vi "FeedbackDecode_MSMS2DEKA.vi"(7 "CtrlMode":T1(array[ring])=[enum."Position", enum."Position", enum."Position", enum."Position", enum."Position", enum."Position", enum."Position", enum."Position", enum."Position", enum."Position", enum."Position", enum."Position"], 8 "Sensors":T3={"Position"={"WriRot"=-84.0, "WriPitch"=-163.0, "IndFlex"=3175.0, "MRPFlex"=2598.0, "ThuRawPitch"=2802.0, "ThuRawYaw"=4899.0, "ThuYaw"=1941.0, "ThuPitch"=4899.0}, "Force"={"IndLat"=20.0, "IndTip"=36.0, "MidTip"=27.0, "RinTip"=34.0, "PinkyTip"=24.0, "PalmDist"=57.0, "PalmProx"=68.0, "HandEdge"=25.0, "HandDorsal"=105.0, "ThuUlnar"=15.0, "ThuRadial"=15.0, "ThuTip"=14.0, "ThuDorsal"=21.0}}, 9 "ConnDEKA":bool, 10 "ResetPID":bool, 11 "MSMSMvnt":dbl[](array[numeric])=[0.0, 0.0, 0.0, 0.0, 0.0, 0.0, 0.0, 0.0, 0.0, 0.0, 0.0, 0.0] min=-1.0 max=1.0) -> (0 "ACIOut":T4[](array[typedef])=[{"Timestamp"=0.0, "ArbitrationId"=528, "IsRemote"=0, "DataLength"=8, "Data"=[0, 0, 0, 0, 0, 38, 0, 0]}, {"Timestamp"=0.0, "ArbitrationId"=529, "IsRemote"=0, "DataLength"=8, "Data"=[0, 0, 0, 52, 0, 50, 0, 0]}, {"Timestamp"=0.0, "ArbitrationId"=530, "IsRemote"=0, "DataLength"=8, "Data"=[0, 26, 0, 0, 0, 0, 0, 47]}, {"Timestamp"=0.0, "ArbitrationId"=531, "IsRemote"=0, "DataLength"=8, "Data"=[0, 0, 0, 0, 0, 0, 0, 0]}] {"Data" format="%.0x"; "ArbitrationId" format="%.0x"; "Timestamp" format="%<%I:%M:%S%3u %p\n%m/%d/%Y>T"})   [LabVIEW 2020]
uses:
  <vilib>/nican/nican.llb/CanFrameTimed.ctl
  <vilib>/addons/control/pid/pid.llb/PID Advanced (DBL Array).vi
  <vilib>/addons/control/pid/pid.llb/PID Parameter Manager (DBL Array).vi
  <vilib>/addons/control/pid/pid.llb/PID Derivative Action Buffered (DBL Array).vi
  <vilib>/addons/control/pid/pid.llb/PID Get Advanced Error (DBL Array).vi
  <vilib>/addons/control/pid/pid.llb/PID Integral Action Buffered (DBL Array).vi
  <vilib>/addons/control/pid/pid.llb/PID Resize 1D Array.vi
  <vilib>/addons/control/pid/pid.llb/PID Get Advanced Error (DBL).vi
  FeedbackDecode_Globals.vi
  <vilib>/addons/control/pid/pid.llb/PID Output Rate Limiter (DBL Array).vi
  <vilib>/addons/control/pid/NI_PID_pid.lvlib
panel:
  in  "HandType":enum16{"Left", "Right"}(ring)=enum."Right"
  in  "SetPoint":dbl[](array[numeric])=[0.85, 0.35, 0.35, 0.35, 0.0, 0.0]
  in  "RmThresh":dbl
  in  "ThuMin":dbl=4000.0
  in  "ThuMax":dbl=5800.0
  in  "linearity":dbl=1.0 format="%.2f"
  in  "outputrate":dbl=3000.0 format="%.2f"
  in  "PIDGains":T2(array[cluster])=[{"proportional gain (Kc)"=0.5, "integral time (Ti, min)"=0.0, "derivative time (Td, min)"=0.0}, {"proportional gain (Kc)"=1.0, "integral time (Ti, min)"=0.0, "derivative time (Td, min)"=0.0}, {"proportional gain (Kc)"=1.0, "integral time (Ti, min)"=0.0, "derivative time (Td, min)"=0.0}, {"proportional gain (Kc)"=1.0, "integral time (Ti, min)"=0.0, "derivative time (Td, min)"=0.0}, {"proportional gain (Kc)"=3.0, "integral time (Ti, min)"=0.0, "derivative time (Td, min)"=0.0}, {"proportional gain (Kc)"=3.0, "integral time (Ti, min)"=0.0, "derivative time (Td, min)"=0.0}] {"derivative time (Td, min)" format="%.5f"; "integral time (Ti, min)" format="%.5f"; "proportional gain (Kc)" format="%.5f"}
  in  "ACIInit":T4[](array[typedef])=[{"Timestamp"=0.0, "ArbitrationId"=528, "IsRemote"=0, "DataLength"=8, "Data"=[0, 0, 0, 0, 0, 0, 0, 0]}, {"Timestamp"=0.0, "ArbitrationId"=529, "IsRemote"=0, "DataLength"=8, "Data"=[0, 0, 0, 0, 0, 0, 0, 0]}, {"Timestamp"=0.0, "ArbitrationId"=530, "IsRemote"=0, "DataLength"=8, "Data"=[0, 0, 0, 0, 0, 0, 0, 0]}, {"Timestamp"=0.0, "ArbitrationId"=531, "IsRemote"=0, "DataLength"=8, "Data"=[0, 0, 0, 0, 0, 0, 0, 0]}] {"Data" format="%.0x"; "ArbitrationId" format="%.0x"; "Timestamp" format="%<%I:%M:%S%3u %p\n%m/%d/%Y>T"}
  # "ThuLimit of 5800 aligns with index,\n~6000 for tripod."
  # "ThuPitch"
  # "Thumb"
  # "Index"
  # "Middle"
  # "ThuYaw"
  # "Ring"
  # "Little"
  # "ThumbInt"
  # "ThuPitchUp"
  # "IndFlex"
  # "IndexInt"
  # "ThuPitchDown"
  # "Ring Int"
  # "ThuYawRight"
  # "Little Int"
  # "ThuYawLeft"
  # "WristPitch"
  # "MRPFlex"
  # "WristYaw"
  # "IndFlex"
  # "WristRoll"
  # "IndExt"
  # "WriRot"
  # "MRPFlex"
  # "MRPExt"
  # "WriPitch"
  # "WriPronate"
  # "WriSupinate"
  # "WriExt"
  # "WriFlex"
  # "ModeSelect"
  # "N/A"
  # "N/A"
  # "N/A"
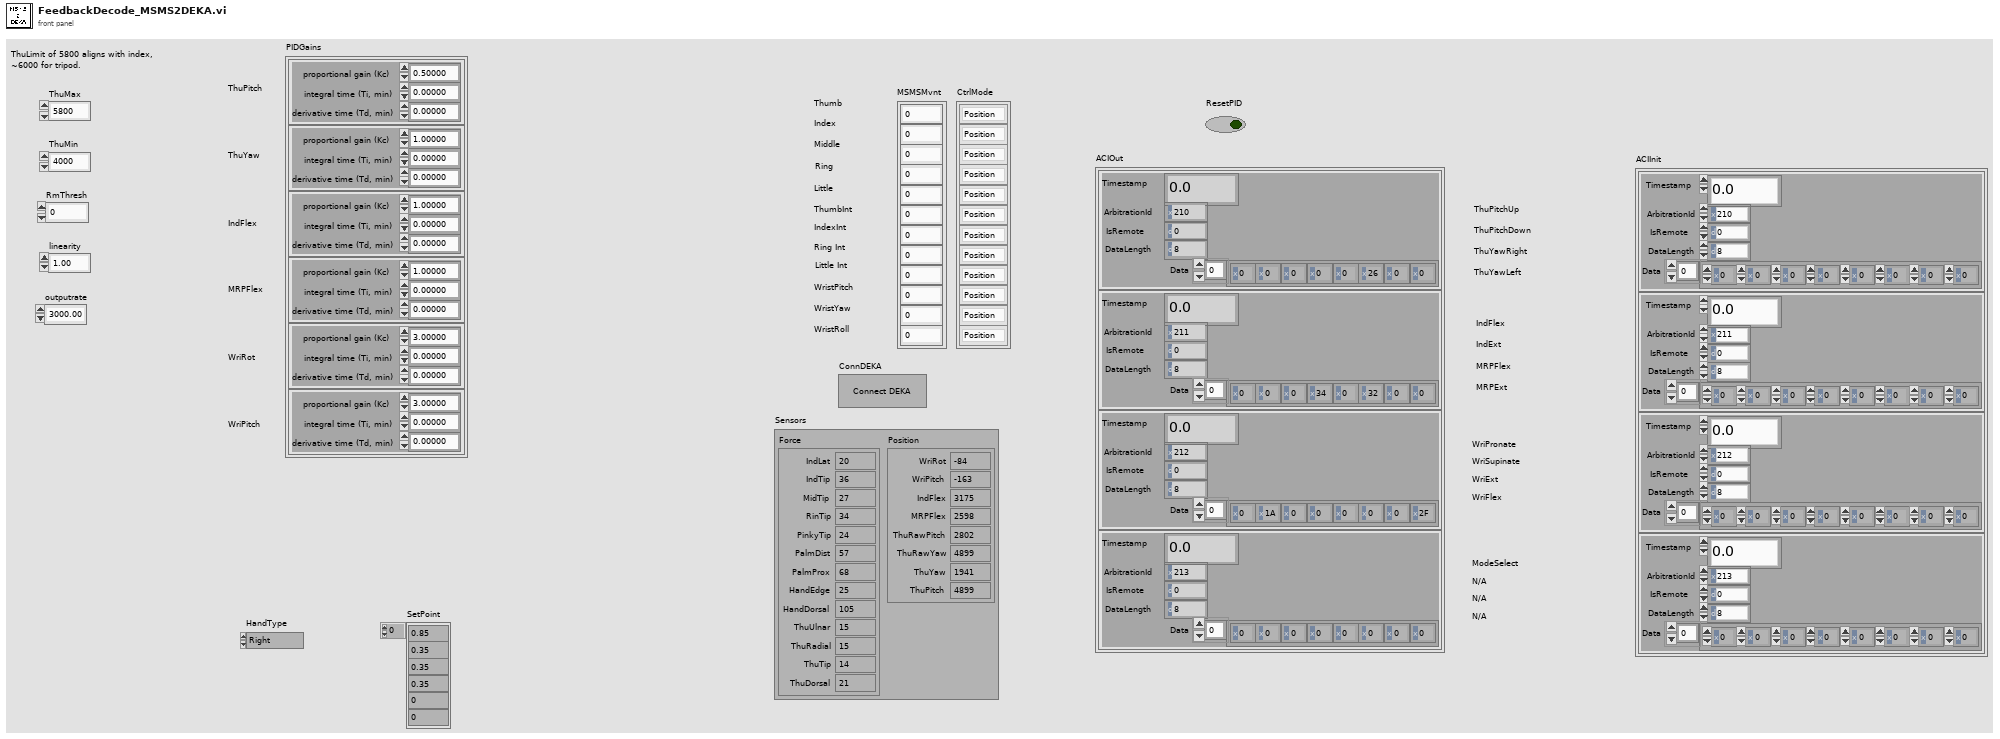
[diagram p1: front panel]
types:
  T1 = enum16{"Position", "Latching", "Leaky", "Velocity"}[]
  T2 = cluster{"proportional gain (Kc)":dbl, "integral time (Ti, min)":dbl, "derivative time (Td, min)":dbl}[]
  T3 = cluster{"Position":cluster{"WriRot":dbl, "WriPitch":dbl, "IndFlex":dbl, "MRPFlex":dbl, "ThuRawPitch":dbl, "ThuRawYaw":dbl, "ThuYaw":dbl, "ThuPitch":dbl}, "Force":cluster{"IndLat":dbl, "IndTip":dbl, "MidTip":dbl, "RinTip":dbl, "PinkyTip":dbl, "PalmDist":dbl, "PalmProx":dbl, "HandEdge":dbl, "HandDorsal":dbl, "ThuUlnar":dbl, "ThuRadial":dbl, "ThuTip":dbl, "ThuDorsal":dbl}}
  T4 = typedef "CanFrameTimed.ctl" = cluster{"Timestamp":dbl, "ArbitrationId":u32, "IsRemote":u8, "DataLength":u8, "Data":u8[]}
  T5 = cluster{"setpoint high":dbl, "setpoint low":dbl}[]
  T6 = enum16{"Position", "Latching", "Leaky", "Velocity"}
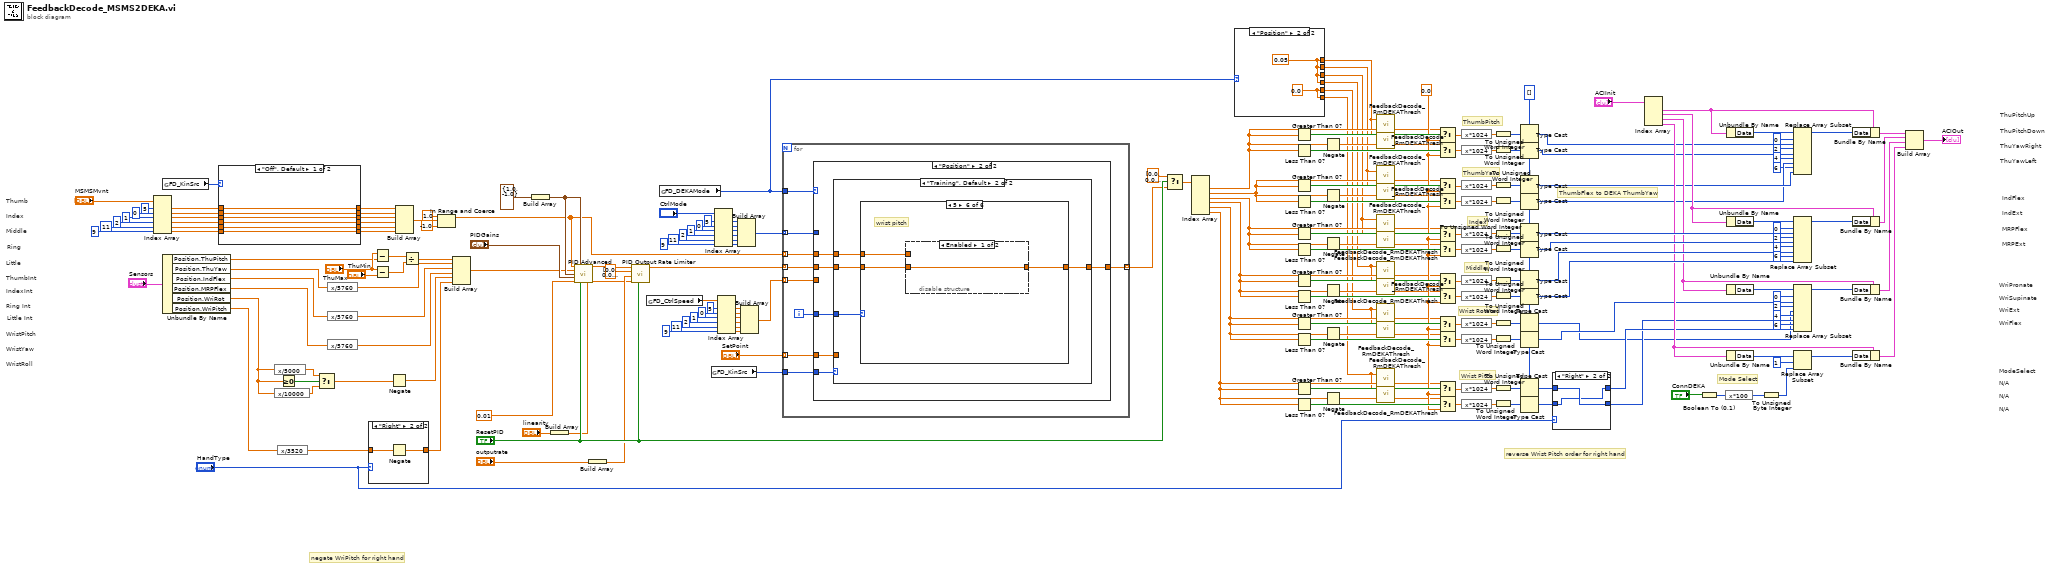
[diagram p0: block diagram]
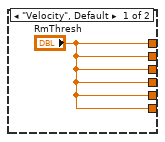
[diagram p4: hidden frame]
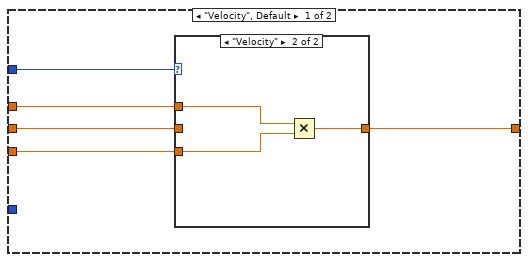
[diagram p5: hidden frame]
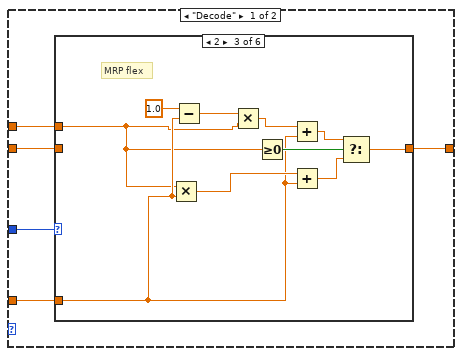
[diagram p7: hidden frame]
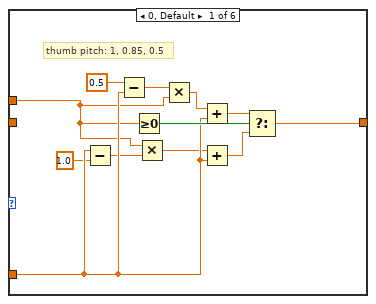
[diagram p8: hidden frame]
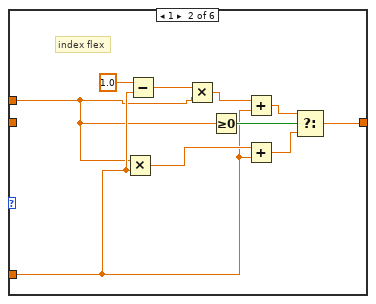
[diagram p9: hidden frame]
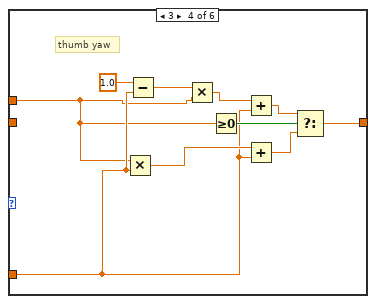
[diagram p10: hidden frame]
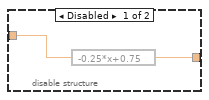
[diagram p14: hidden frame]
diagram:
  w144 = u8[] []
  w86 = 0.0
  # "reverse Wrist Pitch order for right hand"
  # "negate WriPitch for right hand"
  # "ThumbPitch"
  # "N/A"
  # "N/A"
  # "N/A"
  # "ModeSelect"
  # "WriFlex"
  # "WriExt"
  # "WriSupinate"
  # "WriPronate"
  # "MRPExt"
  # "MRPFlex"
  # "IndExt"
  # "IndFlex"
  # "ThuYawLeft"
  # "ThuYawRight"
  # "ThuPitchDown"
  # "ThuPitchUp"
  # "ThumbFlex to DEKA ThumbYaw"
  # "Mode Select"
  # "Wrist Pitch"
  # "Wrist Rotate"
  # "Middle"
  # "Index"
  # "ThumbYaw"
  # "Little Int"
  # "WristRoll"
  # "WristYaw"
  # "WristPitch"
  # "Ring Int"
  # "IndexInt"
  # "ThumbInt"
  # "Little"
  # "Ring"
  # "Middle"
  # "Index"
  # "Thumb"
  n1 = Index Array(array="MSMSMvnt", index #1=5 ("index"), index #2=0 ("index"), index #3=1 ("index"), index #4=2 ("index"), index #5=11 ("index"), index #6=9 ("index")) -> (element #1=w60:dbl, element #2=w59:dbl, element #3=w58:dbl, element #4=w57:dbl, element #5=w56:dbl, element #6=w55:dbl)
  n2 = global read "FeedbackDecode_Globals.vi" "FD_KinSrc"() -> (w61:enum16{"Off", "Training", "Decode", "COB"})
  n3 = Unbundle By Name("Sensors") -> ("Position.ThuPitch"=w95:dbl, "Position.ThuYaw"=w133:dbl, "Position.IndFlex"=w132:dbl, "Position.MRPFlex"=w131:dbl, "Position.WriRot"=w106:dbl, "Position.WriPitch"=w5:dbl)
  n4 = case shown="\"Off\", Default" w61 {
    tunnel: w60 -> [w230 w238]
    tunnel: w59 -> [w229 w236]
    tunnel: w58 -> [w228 w234]
    tunnel: w57 -> [w227 w232]
    tunnel: w56 -> [w226 w240]
    tunnel: w55 -> [w225 w239]
    tunnel: [w230 w237] -> w54
    tunnel: [w229 w235] -> w53
    tunnel: [w228 w233] -> w52
    tunnel: [w227 w231] -> w51
    tunnel: [w226 w240] -> w50
    tunnel: [w225 w239] -> w49
    frame "Off", Default {
    }
    frame "Training" {
      n5 = expression code="x*0.5+0.5"(w238) -> (w237:dbl)
      n6 = expression code="x*0.5+0.3"(w236) -> (w235:dbl)
      n7 = expression code="x*0.5+0.5"(w234) -> (w233:dbl)
      n8 = expression code="x*0.5+0.5"(w232) -> (w231:dbl)
    }
  }
  n9 = expression code="x/5000"(w106) -> (w108:dbl)
  n10 = expression code="x/10000"(w106) -> (w107:dbl)
  n11 = expression code="x/3520"(w5) -> (w4:dbl)
  n12 = Greater Or Equal To 0?(x=w106) -> (x >= 0?=w109:bool)
  n13 = Select(t=w108, s=w109, f=w107) -> (s? t:f=w3:dbl)
  n14 = expression code="x/5760"(w133) -> (w103:dbl)
  n15 = expression code="x/5760"(w132) -> (w102:dbl)
  n16 = expression code="x/5760"(w131) -> (w101:dbl)
  n17 = case shown="\"Right\"" "HandType" {
    tunnel: w4 -> [w241 w242]
    tunnel: [w241 w243] -> w100
    frame "Left", Default {
    }
    frame "Right" {
      n18 = Negate(x=w242) -> (-x=w243:dbl)
    }
  }
  n19 = Subtract(x="ThuMax", y=w95) -> (x-y=w97:dbl)
  n20 = Subtract(x="ThuMax", y="ThuMin") -> (x-y=w96:dbl)
  n21 = Negate(x=w3) -> (-x=w2:dbl)
  n22 = Build Array(w54, w53, w52, w51, w50, w49) -> (w123:dbl[])
  n23 = Divide(x=w97, y=w96) -> (x/y=w94:dbl)
  n24 = In Range and Coerce(upper limit=1.0, x=w123, lower limit=-1.0) -> (coerced(x)=w110:dbl[])  [unwired: 1 out]
  n25 = Build Array(w94, w103, w102, w101, w2, w100) -> (w99:dbl[])
  n26 = Build Array(cluster{"setpoint high":dbl, "setpoint low":dbl} {"setpoint high"=1.0, "setpoint low"=-1.0} ("setpoint range")) -> (w113:T5)
  n27 = Build Array("linearity") -> (w114:dbl[])
  n28 = call-poly <vilib>:"PID Advanced.vi"("setpoint"=w110, "output range"=w113, "process variable"=w99, "setpoint range"=w113, "PID gains"="PIDGains", "dt (s)"=0.01, "reinitialize? (F)"="ResetPID", "linearity"=w114) -> ("output"=w119:dbl[], "dt out (s)"=w116:dbl)  [unwired: 6 in]
  n29 = Build Array("outputrate") -> (w117:dbl[])
  n30 = call-poly <vilib>:"PID Output Rate Limiter.vi"("reinitialize? (F)"="ResetPID", "dt (s)"=w116, "output rate (EGU/min)"=w117, "initial output"=dbl[] [0.0, 0.0, 0.0, 0.0, 0.0, 0.0], "input (controller output)"=w119) -> ("output"=w112:dbl[])  [unwired: 3 in, 1 out]
  n31 = global read "FeedbackDecode_Globals.vi" "FD_CtrlSpeed"() -> (w22:sgl[])
  n32 = global read "FeedbackDecode_Globals.vi" "FD_DEKAMode"() -> (w20:enum16{"Velocity", "Position"})
  n33 = global read "FeedbackDecode_Globals.vi" "FD_KinSrc"() -> (w13:enum16{"Off", "Training", "Decode", "COB"})
  n34 = Index Array(array="CtrlMode", index #1=5 ("index"), index #2=0 ("index"), index #3=1 ("index"), index #4=2 ("index"), index #5=11 ("index"), index #6=9 ("index")) -> (element #1=w41:T6, element #2=w40:T6, element #3=w39:T6, element #4=w38:T6, element #5=w37:T6, element #6=w36:T6)
  n35 = Index Array(array=w22, index #1=5 ("index"), index #2=0 ("index"), index #3=1 ("index"), index #4=2 ("index"), index #5=11 ("index"), index #6=9 ("index")) -> (element #1=w29:sgl, element #2=w30:sgl, element #3=w31:sgl, element #4=w32:sgl, element #5=w33:sgl, element #6=w34:sgl)
  n36 = Build Array(w41, w40, w39, w38, w37, w36) -> (w35:T1)
  n37 = Build Array(w29, w30, w31, w32, w33, w34) -> (w21:sgl[])
  n38 = for {
    tunnel: w112 -> [w252] mode=indexing
    tunnel: [w251] -> w111 mode=indexing
    tunnel: w110 -> [w250] mode=indexing
    tunnel: w35 -> [w249] mode=indexing
    tunnel: w21 -> [w248] mode=indexing
    tunnel: w20 -> [w247]
    tunnel: w13 -> [w245]
    tunnel: "SetPoint" -> [w244] mode=indexing
    i -> [w246]
    n39 = case shown="\"Position\"" w247 {
      tunnel: w252 -> [w257 w264]
      tunnel: [w256 w265] -> w251
      tunnel: w250 -> [w255 w266]
      tunnel: w249 -> [w254 _]
      tunnel: w248 -> [w253 _]
      tunnel: w246 -> [_ w267]
      tunnel: w245 -> [_ w263]
      tunnel: w244 -> [_ w262]
      frame "Velocity", Default {
        n40 = case shown="\"Velocity\"" w254 {
          tunnel: w257 -> [w258 _]
          tunnel: [w258 w260] -> w256
          tunnel: w255 -> [_ w261]
          tunnel: w253 -> [_ w259]
          frame "Position", Default {
          }
          frame "Velocity" {
            n41 = Multiply(x=w261, y=w259) -> (x*y=w260:dbl)
          }
        }
      }
      frame "Position" {
        n42 = case shown="\"Training\", Default" w263 {
          tunnel: w267 -> [w272 w317]
          tunnel: w266 -> [w271 w320]
          tunnel: [w270 w319] -> w265
          tunnel: w264 -> [w269 w318]
          tunnel: w262 -> [w268 _]
          frame "Decode" {
            n43 = case shown="2" w272 {
              tunnel: w271 -> [w274 w286 w296 w306 _ _]
              tunnel: [w283 w293 w303 w313 w315 w316] -> w270
              tunnel: w269 -> [_ _ _ _ w315 w316]
              tunnel: w268 -> [w277 w288 w298 w308 _ _]
              frame 0, Default {
                # "thumb pitch: 1, 0.85, 0.5"
                n44 = Subtract(x=w277, y=1.0) -> (x-y=w275:dbl)
                n45 = Subtract(x=0.5, y=w277) -> (x-y=w279:dbl)
                n46 = Greater Or Equal To 0?(x=w274) -> (x >= 0?=w284:bool)
                n47 = Multiply(x=w274, y=w275) -> (x*y=w273:dbl)
                n48 = Multiply(x=w279, y=w274) -> (x*y=w278:dbl)
                n49 = Add(x=w278, y=w277) -> (x+y=w281:dbl)
                n50 = Add(x=w273, y=w277) -> (x+y=w282:dbl)
                n51 = Select(t=w281, s=w284, f=w282) -> (s? t:f=w283:dbl)
              }
              frame 1 {
                # "index flex"
                n52 = Multiply(x=w286, y=w288) -> (x*y=w290:dbl)
                n53 = Subtract(x=1.0, y=w288) -> (x-y=w287:dbl)
                n54 = Multiply(x=w287, y=w286) -> (x*y=w285:dbl)
                n55 = Greater Or Equal To 0?(x=w286) -> (x >= 0?=w294:bool)
                n56 = Add(x=w285, y=w288) -> (x+y=w292:dbl)
                n57 = Add(x=w290, y=w288) -> (x+y=w291:dbl)
                n58 = Select(t=w292, s=w294, f=w291) -> (s? t:f=w293:dbl)
              }
              frame 2 {
                # "MRP flex"
                n59 = Multiply(x=w296, y=w298) -> (x*y=w300:dbl)
                n60 = Subtract(x=1.0, y=w298) -> (x-y=w297:dbl)
                n61 = Multiply(x=w297, y=w296) -> (x*y=w295:dbl)
                n62 = Greater Or Equal To 0?(x=w296) -> (x >= 0?=w304:bool)
                n63 = Add(x=w295, y=w298) -> (x+y=w302:dbl)
                n64 = Add(x=w300, y=w298) -> (x+y=w301:dbl)
                n65 = Select(t=w302, s=w304, f=w301) -> (s? t:f=w303:dbl)
              }
              frame 3 {
                # "thumb yaw"
                n66 = Multiply(x=w306, y=w308) -> (x*y=w310:dbl)
                n67 = Subtract(x=1.0, y=w308) -> (x-y=w307:dbl)
                n68 = Multiply(x=w307, y=w306) -> (x*y=w305:dbl)
                n69 = Greater Or Equal To 0?(x=w306) -> (x >= 0?=w314:bool)
                n70 = Add(x=w305, y=w308) -> (x+y=w312:dbl)
                n71 = Add(x=w310, y=w308) -> (x+y=w311:dbl)
                n72 = Select(t=w312, s=w314, f=w311) -> (s? t:f=w313:dbl)
              }
              frame 4 {
                # "wrist rotation"
              }
              frame 5 {
                # "wrist pitch"
              }
            }
          }
          frame "Training", Default {
            n73 = case shown="5" w317 {
              tunnel: w320 -> [w322 w326 w327 w328 w329 w334]
              tunnel: [w321 w326 w327 w328 w330 w335] -> w319
              tunnel: w318 -> [_ _ _ _ w331 w336]
              frame 0, Default {
                # "thumb pitch"
                n74 = disable-structure shown="Enabled" {
                  disable-tunnel: w322 -> [w324 w325]
                  disable-tunnel: [w323 w325] -> w321
                  frame Disabled {
                    n75 = expression code="-0.25*x+0.75"(w324) -> (w323:dbl)
                  }
                  frame Enabled {
                  }
                }
              }
              frame 1 {
                # "thumb yaw"
              }
              frame 2 {
                # "Index Flex"
              }
              frame 3 {
                # "MRP Flex"
              }
              frame 4 {
                # "wrist rotation"
                n76 = disable-structure shown="Enabled" {
                  disable-tunnel: w331 -> [w332 _]
                  disable-tunnel: [w332 w333] -> w330
                  disable-tunnel: w329 -> [_ w333]
                  frame Disabled {
                  }
                  frame Enabled {
                  }
                }
              }
              frame 5 {
                # "wrist pitch"
                n77 = disable-structure shown="Enabled" {
                  disable-tunnel: w336 -> [w337 _]
                  disable-tunnel: [w337 w338] -> w335
                  disable-tunnel: w334 -> [_ w338]
                  frame Enabled {
                  }
                  frame Disabled {
                  }
                }
              }
            }
          }
        }
      }
    }
  }
  n78 = Select(t=dbl[] [0.0, 0.0, 0.0, 0.0, 0.0, 0.0], s="ResetPID", f=w111) -> (s? t:f=w128:dbl[])
  n79 = Index Array(array=w128) -> (element #1=w85:dbl, element #2=w81:dbl, element #3=w77:dbl, element #4=w73:dbl, element #5=w69:dbl, element #6=w65:dbl)  [unwired: 6 in]
  n80 = case shown="\"Position\"" w20 {
    tunnel: ["RmThresh" w341] -> w19
    tunnel: ["RmThresh" w341] -> w18
    tunnel: ["RmThresh" w341] -> w17
    tunnel: ["RmThresh" w341] -> w16
    tunnel: ["RmThresh" w340] -> w15
    tunnel: ["RmThresh" w340] -> w14
    frame "Velocity", Default {
    }
    frame "Position" {
      w340 = 0.0 ("RmThresh")
      w341 = 0.05 ("RmThresh")
    }
  }
  n81 = Greater Than 0?(x=w85) -> (x > 0?=w129:bool)
  n82 = Less Than 0?(x=w85) -> (x < 0?=w92:bool)
  n83 = Greater Than 0?(x=w81) -> (x > 0?=w212:bool)
  n84 = Less Than 0?(x=w81) -> (x < 0?=w91:bool)
  n85 = Greater Than 0?(x=w77) -> (x > 0?=w223:bool)
  n86 = Less Than 0?(x=w77) -> (x < 0?=w90:bool)
  n87 = Greater Than 0?(x=w73) -> (x > 0?=w186:bool)
  n88 = Less Than 0?(x=w73) -> (x < 0?=w89:bool)
  n89 = Greater Than 0?(x=w69) -> (x > 0?=w176:bool)
  n90 = Less Than 0?(x=w69) -> (x < 0?=w88:bool)
  n91 = Greater Than 0?(x=w65) -> (x > 0?=w163:bool)
  n92 = Less Than 0?(x=w65) -> (x < 0?=w87:bool)
  n93 = Negate(x=w85) -> (-x=w83:dbl)
  n94 = Negate(x=w81) -> (-x=w79:dbl)
  n95 = Negate(x=w77) -> (-x=w75:dbl)
  n96 = Negate(x=w73) -> (-x=w71:dbl)
  n97 = Negate(x=w69) -> (-x=w67:dbl)
  n98 = Negate(x=w65) -> (-x=w63:dbl)
  n99 = call "FeedbackDecode_RmDEKAThresh.vi"("ValIn"=w85, "Thresh"=w19) -> ("ValOut"=w84:dbl)  [unwired: 1 in]
  n100 = call "FeedbackDecode_RmDEKAThresh.vi"("ValIn"=w83, "Thresh"=w19) -> ("ValOut"=w82:dbl)  [unwired: 1 in]
  n101 = call "FeedbackDecode_RmDEKAThresh.vi"("ValIn"=w81, "Thresh"=w18) -> ("ValOut"=w80:dbl)  [unwired: 1 in]
  n102 = call "FeedbackDecode_RmDEKAThresh.vi"("ValIn"=w79, "Thresh"=w18) -> ("ValOut"=w78:dbl)  [unwired: 1 in]
  n103 = call "FeedbackDecode_RmDEKAThresh.vi"("ValIn"=w77, "Thresh"=w17) -> ("ValOut"=w76:dbl)  [unwired: 1 in]
  n104 = call "FeedbackDecode_RmDEKAThresh.vi"("ValIn"=w75, "Thresh"=w17) -> ("ValOut"=w74:dbl)  [unwired: 1 in]
  n105 = call "FeedbackDecode_RmDEKAThresh.vi"("ValIn"=w73, "Thresh"=w16) -> ("ValOut"=w72:dbl)  [unwired: 1 in]
  n106 = call "FeedbackDecode_RmDEKAThresh.vi"("ValIn"=w71, "Thresh"=w16) -> ("ValOut"=w70:dbl)  [unwired: 1 in]
  n107 = call "FeedbackDecode_RmDEKAThresh.vi"("ValIn"=w69, "Thresh"=w15) -> ("ValOut"=w68:dbl)  [unwired: 1 in]
  n108 = call "FeedbackDecode_RmDEKAThresh.vi"("ValIn"=w67, "Thresh"=w15) -> ("ValOut"=w66:dbl)  [unwired: 1 in]
  n109 = call "FeedbackDecode_RmDEKAThresh.vi"("ValIn"=w65, "Thresh"=w14) -> ("ValOut"=w64:dbl)  [unwired: 1 in]
  n110 = call "FeedbackDecode_RmDEKAThresh.vi"("ValIn"=w63, "Thresh"=w14) -> ("ValOut"=w62:dbl)  [unwired: 1 in]
  n111 = Select(t=w84, s=w129, f=w86) -> (s? t:f=w148:dbl)
  n112 = Select(t=w82, s=w92, f=w86) -> (s? t:f=w147:dbl)
  n113 = Select(t=w80, s=w212, f=w86) -> (s? t:f=w213:dbl)
  n114 = Select(t=w78, s=w91, f=w86) -> (s? t:f=w214:dbl)
  n115 = Select(t=w76, s=w223, f=w86) -> (s? t:f=w222:dbl)
  n116 = Select(t=w74, s=w90, f=w86) -> (s? t:f=w221:dbl)
  n117 = Select(t=w72, s=w186, f=w86) -> (s? t:f=w187:dbl)
  n118 = Select(t=w70, s=w89, f=w86) -> (s? t:f=w188:dbl)
  n119 = Select(t=w68, s=w176, f=w86) -> (s? t:f=w175:dbl)
  n120 = Select(t=w66, s=w88, f=w86) -> (s? t:f=w174:dbl)
  n121 = Select(t=w64, s=w163, f=w86) -> (s? t:f=w164:dbl)
  n122 = Select(t=w62, s=w87, f=w86) -> (s? t:f=w165:dbl)
  n123 = expression code="x*1024"(w148) -> (w146:dbl)
  n124 = expression code="x*1024"(w147) -> (w145:dbl)
  n125 = expression code="x*1024"(w213) -> (w215:dbl)
  n126 = expression code="x*1024"(w214) -> (w216:dbl)
  n127 = expression code="x*1024"(w222) -> (w220:dbl)
  n128 = expression code="x*1024"(w221) -> (w219:dbl)
  n129 = expression code="x*1024"(w187) -> (w189:dbl)
  n130 = expression code="x*1024"(w188) -> (w190:dbl)
  n131 = expression code="x*1024"(w175) -> (w173:dbl)
  n132 = expression code="x*1024"(w174) -> (w172:dbl)
  n133 = expression code="x*1024"(w164) -> (w166:dbl)
  n134 = expression code="x*1024"(w165) -> (w167:dbl)
  n135 = To Unsigned Word Integer(number=w146) -> (unsigned 16bit integer=w149:u16)
  n136 = To Unsigned Word Integer(number=w145) -> (unsigned 16bit integer=w150:u16)
  n137 = To Unsigned Word Integer(number=w215) -> (unsigned 16bit integer=w211:u16)
  n138 = To Unsigned Word Integer(number=w216) -> (unsigned 16bit integer=w210:u16)
  n139 = To Unsigned Word Integer(number=w220) -> (unsigned 16bit integer=w218:u16)
  n140 = To Unsigned Word Integer(number=w219) -> (unsigned 16bit integer=w217:u16)
  n141 = To Unsigned Word Integer(number=w189) -> (unsigned 16bit integer=w191:u16)
  n142 = To Unsigned Word Integer(number=w190) -> (unsigned 16bit integer=w192:u16)
  n143 = To Unsigned Word Integer(number=w173) -> (unsigned 16bit integer=w171:u16)
  n144 = To Unsigned Word Integer(number=w172) -> (unsigned 16bit integer=w170:u16)
  n145 = To Unsigned Word Integer(number=w166) -> (unsigned 16bit integer=w168:u16)
  n146 = To Unsigned Word Integer(number=w167) -> (unsigned 16bit integer=w169:u16)
  n147 = Type Cast(type=w144, x=w149) -> (*(type *) &x=w105:u8[])
  n148 = Type Cast(type=w144, x=w150) -> (*(type *) &x=w104:u8[])
  n149 = Type Cast(type=w144, x=w211) -> (*(type *) &x=w143:u8[])
  n150 = Type Cast(type=w144, x=w210) -> (*(type *) &x=w142:u8[])
  n151 = Type Cast(type=w144, x=w218) -> (*(type *) &x=w195:u8[])
  n152 = Type Cast(type=w144, x=w217) -> (*(type *) &x=w193:u8[])
  n153 = Type Cast(type=w144, x=w191) -> (*(type *) &x=w185:u8[])
  n154 = Type Cast(type=w144, x=w192) -> (*(type *) &x=w184:u8[])
  n155 = Type Cast(type=w144, x=w171) -> (*(type *) &x=w6:u8[])
  n156 = Type Cast(type=w144, x=w170) -> (*(type *) &x=w7:u8[])
  n157 = Type Cast(type=w144, x=w168) -> (*(type *) &x=w11:u8[])
  n158 = Type Cast(type=w144, x=w169) -> (*(type *) &x=w9:u8[])
  n159 = case shown="\"Right\"" "HandType" {
    tunnel: w11 -> [w343 w345]
    tunnel: [w343 w344] -> w10
    tunnel: w9 -> [w342 w344]
    tunnel: [w342 w345] -> w8
    frame "Left", Default {
    }
    frame "Right" {
    }
  }
  n160 = Index Array(array="ACIInit") -> (element #1=w204:T4, element #2=w201:T4, element #3=w183:T4, element #4=w159:T4)  [unwired: 4 in]
  n161 = Boolean To (0,1)(Boolean="ConnDEKA") -> (0, 1=w156:i16)
  n162 = expression code="x*100"(w156) -> (w155:i16)
  n163 = Unbundle By Name(w204) -> ("Data"=w203:u8[])
  n164 = Unbundle By Name(w201) -> ("Data"=w198:u8[])
  n165 = Unbundle By Name(w183) -> ("Data"=w178:u8[])
  n166 = Unbundle By Name(w159) -> ("Data"=w161:u8[])
  n167 = To Unsigned Byte Integer(number=w155) -> (unsigned 8bit integer=w154:u8)
  n168 = Replace Array Subset(array=w203, new element #1=w105, index #1=0 ("index"), new element #2=w104, index #2=2 ("index"), new element #3=w142, index #3=4 ("index"), new element #4=w143, index #4=6 ("index")) -> (w202:u8[])
  n169 = Replace Array Subset(array=w198, new element #1=w195, index #1=0 ("index"), new element #2=w193, index #2=2 ("index"), new element #3=w185, index #3=4 ("index"), new element #4=w184, index #4=6 ("index")) -> (w194:u8[])
  n170 = Replace Array Subset(array=w178, new element #1=w7, index #1=0 ("index"), new element #2=w6, index #2=2 ("index"), new element #3=w8, index #3=4 ("index"), new element #4=w10, index #4=6 ("index")) -> (w177:u8[])
  n171 = Replace Array Subset(array=w161, new element=w154, index=1) -> (w162:u8[])
  n172 = Bundle By Name(cluster=w204, "Data"=w202) -> (w209:T4)
  n173 = Bundle By Name(cluster=w201, "Data"=w194) -> (w208:T4)
  n174 = Bundle By Name(cluster=w183, "Data"=w177) -> (w207:T4)
  n175 = Bundle By Name(cluster=w159, "Data"=w162) -> (w158:T4)
  n176 = Build Array(w209, w208, w207, w158) -> (→"ACIOut":T4[])
